vi "Prior_Zmotor_Init.vi"(0 "object in":refnum<class "Prior_Zmotor.lvclass">, 2 "VISA resource name":refnum<visa-resource-name>, 5 "error in (no error)":errorcluster) -> (14 "object out":refnum<class "Prior_Zmotor.lvclass">, 19 "error out":errorcluster)   [LabVIEW 2021, in "Prior_Zmotor.lvclass"]
uses:
  Prior_Zmotor.lvclass
  Prior_Zmotor.lvclass/Prior_Zmotor.ctl
  <vilib>/Instr/_visa.llb/VISA Configure Serial Port (Instr).vi
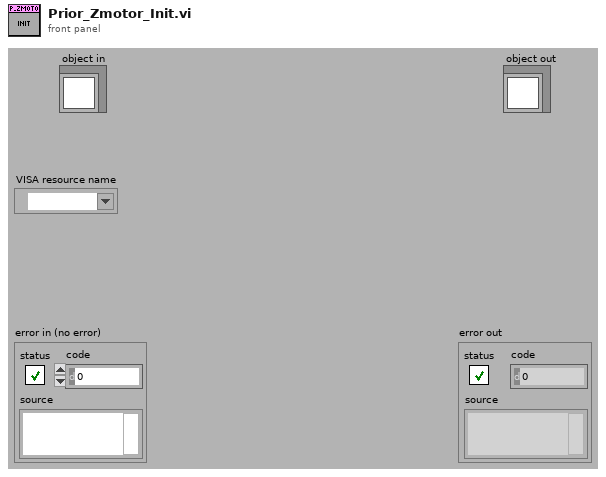
[diagram p1: front panel]
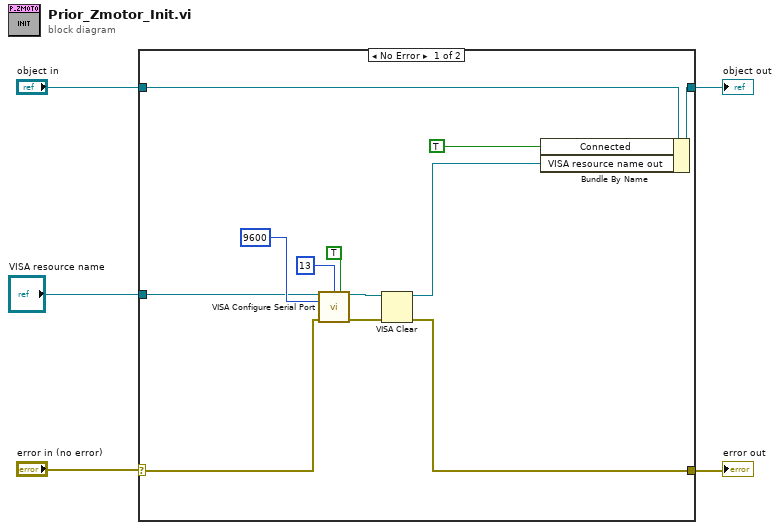
[diagram p0: block diagram]
diagram:
  n1 = case shown="No Error" "error in (no error)" {
    selector: "error in (no error)" -> [w10 w18]
    tunnel: "object in" -> [w17 w19]
    tunnel: [w16 w19] -> w4
    tunnel: [w6 w18] -> w2
    tunnel: "VISA resource name" -> [w11 _]
    frame No Error {
      n2 = call-poly "VISA Configure Serial Port"("VISA resource name"=w11, "termination char\n(0xA = '\\n' = LF)"=u8 13 ("termination char\n(0xA = '\\n' = LF)"), "Enable Termination\nChar (T)"=TRUE ("Enable Termination\nChar (T)"), "baud rate (9600)"=u32 9600, "error in (no error)"=w10) -> ("VISA resource name out"=w9:refnum<visa-resource-name>, "error out"=w7:errorcluster)  [unwired: 9 in]
      n3 = VISA Clear(VISA resource name=w9, error in (no error)=w7) -> (VISA resource name out=w8:refnum<visa-resource-name>, error out=w6:errorcluster)
      n4 = Bundle By Name(cluster=w17, "Connected"=TRUE ("None"), "VISA resource name out"=w8) -> (w16:refnum<class "Prior_Zmotor.lvclass">)
    }
    frame Error {
    }
  }
  "object out" <- w4
  "error out" <- w2
